vi "Create.vi"(8 "error in (no error)":errorcluster, 10 "Input":string) -> (0 "error out":errorcluster, 3 "Network":refnum<class "Network.lvclass">)   [LabVIEW 2020, in "Network.lvclass"]
uses:
  Network.lvclass
  Network.lvclass/Network.ctl
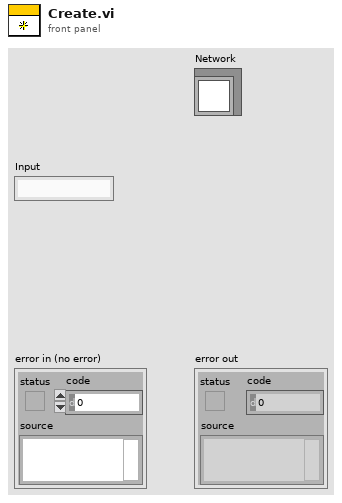
[diagram p1: front panel]
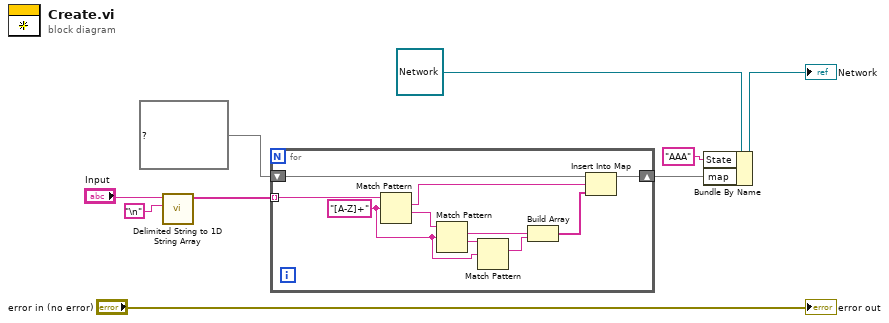
[diagram p0: block diagram]
diagram:
  n1 = call <vilib>:"Delimited String to 1D String Array.vi"("delimiter"="\n", "delimited string"="Input") -> ("string array"=w5:string[])  [unwired: 9 in]
  n2 = for {
    tunnel: w5 -> [w19] mode=indexing
    shift-right: [w13] -> w1
    shift-left: map{string, string[]} {} ("map") -> [w14]
    w10 = "[A-Z]+" ("regular expression")
    n3 = Match Pattern(string=w19, regular expression=w10) -> (match substring=w12:string, after substring=w18:string)  [unwired: 1 in, 2 out]
    n4 = Match Pattern(string=w18, regular expression=w10) -> (match substring=w16:string, after substring=w17:string)  [unwired: 1 in, 2 out]
    n5 = Match Pattern(string=w17, regular expression=w10) -> (match substring=w15:string)  [unwired: 1 in, 3 out]
    n6 = Build Array(w16, w15) -> (w11:string[])
    n7 = Insert Into Map(map in=w14, key=w12, value=w11) -> (map out=w13:map{string, string[]})  [unwired: 2 out]
  }
  n8 = Bundle By Name(cluster=refnum<class "Network.lvclass"> refnum ("Network"), "State"="AAA", "map"=w1) -> (→"Network":refnum<class "Network.lvclass">)
  "error out" <- "error in (no error)"
